vi "Assemble Process Data for Logging.vi"(8 "error in":errorcluster, 10 "Processing loop variables":T1 {"CurrInverter"."last updated" format="%<%H:%M\n%d/%m/%Y>T"; "CurrInverter"."set flag" items=["False", "True"]}) -> (0 "error out":errorcluster, 1 "MeasData":T8, 2 "Processing loop vars out":T1 {"CurrInverter"."last updated" format="%<%H:%M\n%d/%m/%Y>T"; "CurrInverter"."set flag" items=["False", "True"]})   [LabVIEW 2019, in "Main.lvclass"]
doc: "Developed by Kevin Thompson\nkevin@thompsonengineering.net\n\nCopyright 2020\nThompson Engineering, LLC"
uses:
  Main.lvclass
  Common/DataTypes/InverterPhaseData--cluster.ctl
  Common/DataQ_SE/TD MeasData--cluster.ctl
  subvis/DataTypes/averaging variables.ctl
  subvis/DataTypes/ESR alarm variables.ctl
  subvis/DataTypes/Processing loop variables--cluster.ctl
  Common/DataTypes/inverter gain range--cluster.ctl
  Common/DataTypes/inverter offset range--cluster.ctl
  Common/DataTypes/inverter info v2--cluster.ctl
  Common/DataTypes/Inverter database record v2--cluster.ctl
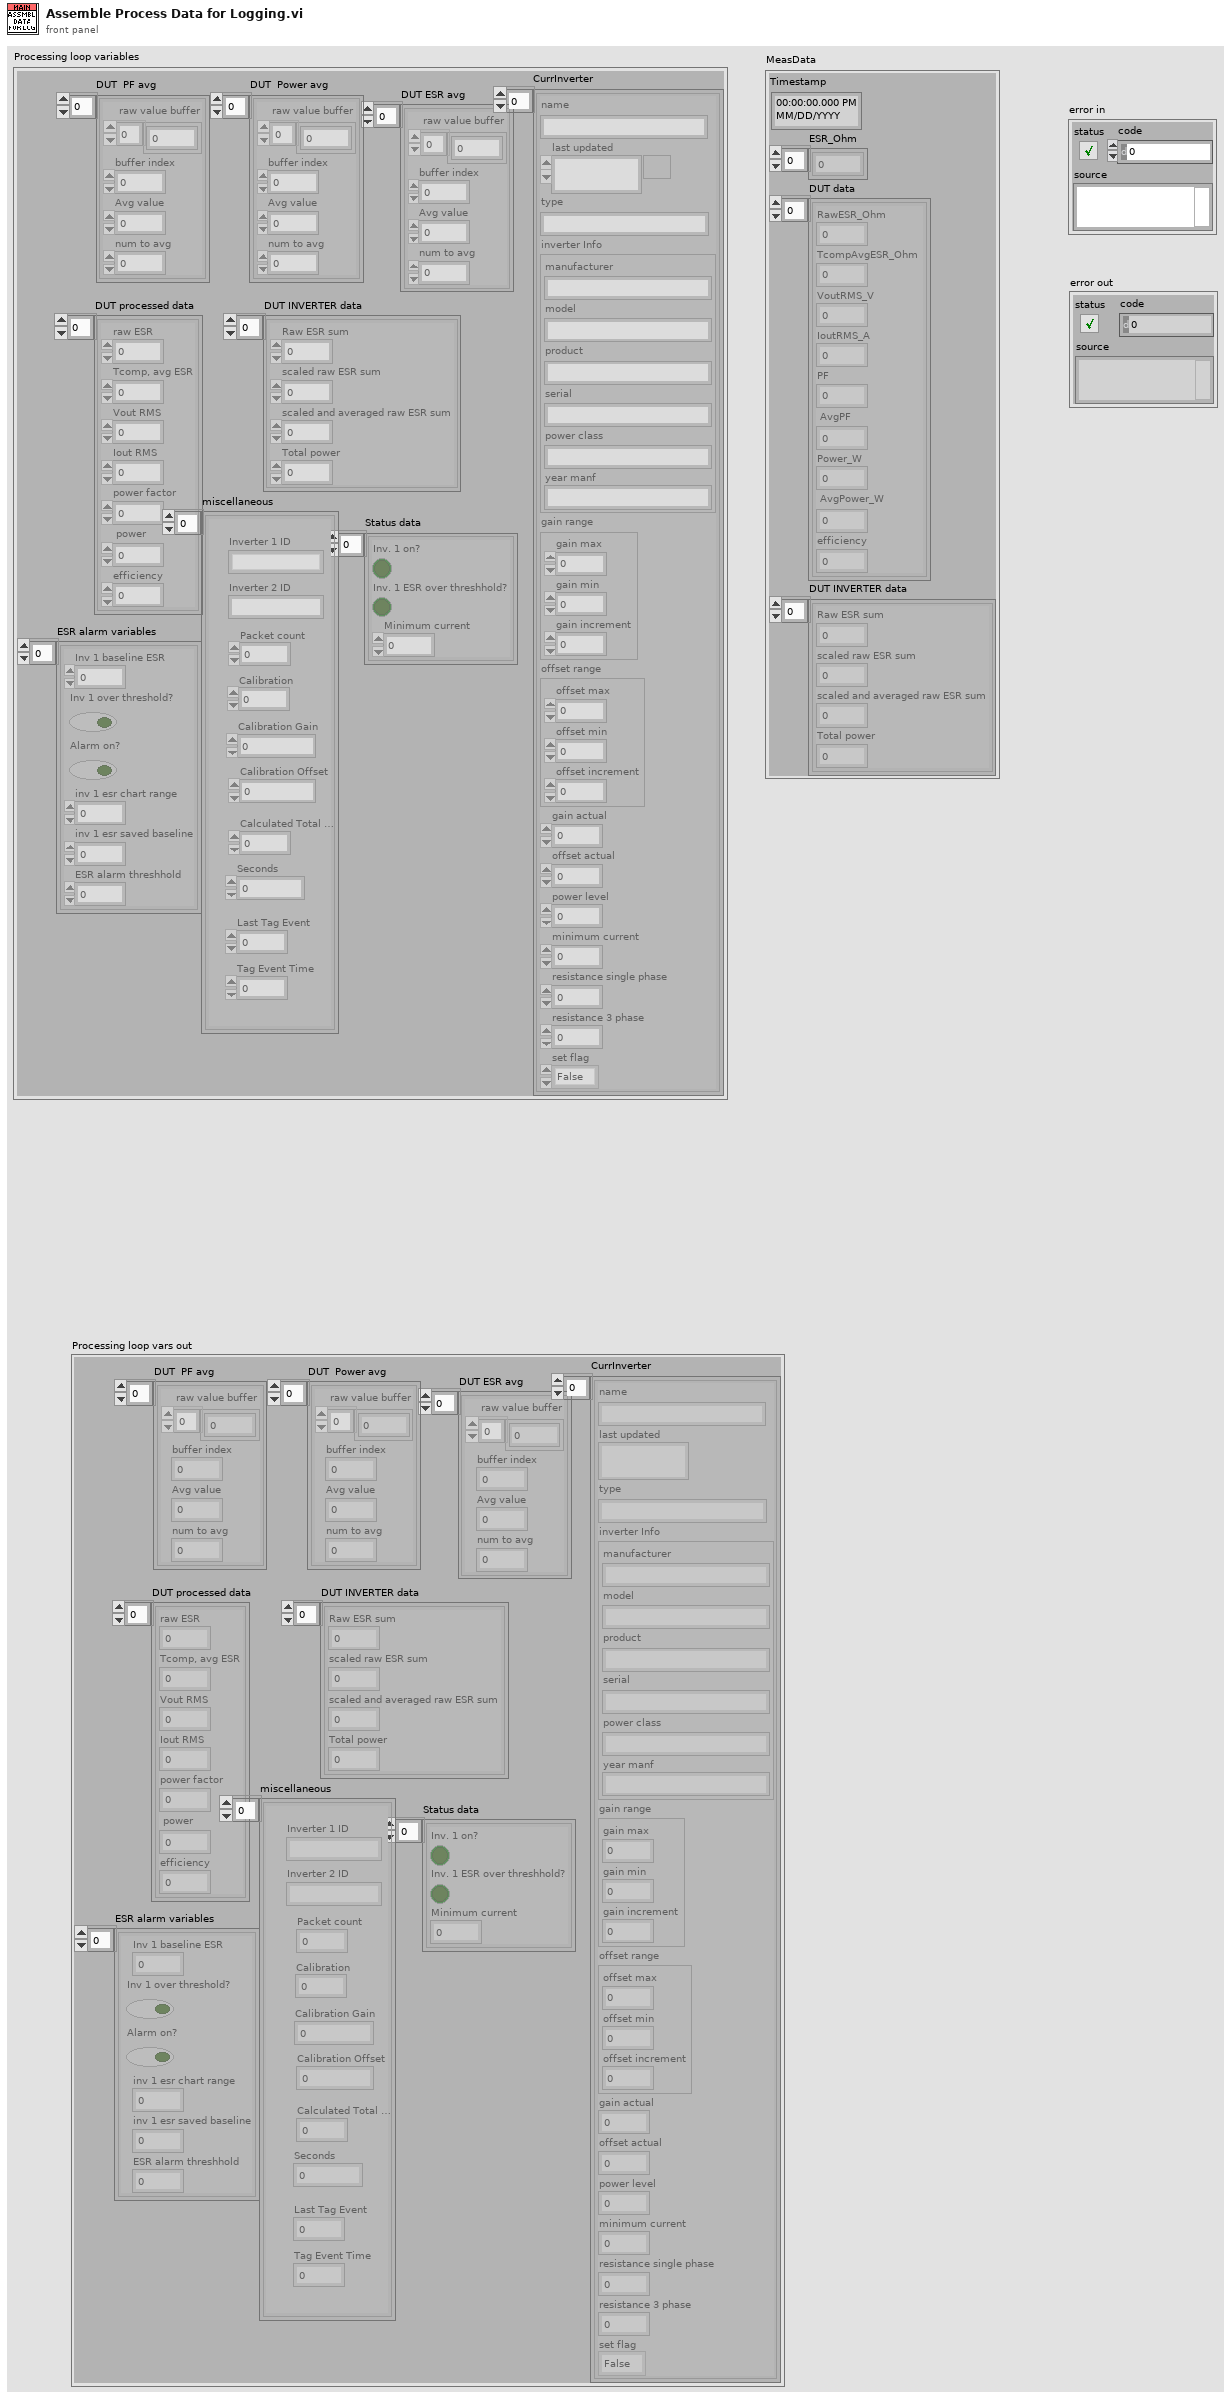
[diagram p1: front panel]
types:
  T1 = typedef "Main.lvclass/Processing loop variables--cluster.ctl" = cluster{"DUT ESR avg":T2[], "DUT  PF avg":T2[], "DUT  Power avg ":T2[], "DUT processed data":cluster{"raw ESR":dbl, "Tcomp, avg ESR":dbl, "Vout RMS":dbl, "Iout RMS":dbl, "power factor":dbl, "power":dbl, "efficiency":dbl}[], "ESR alarm variables":T3[], "Status data":cluster{"Inv. 1 on?":bool, "Inv. 1 ESR over threshhold?":bool, "Minimum current":dbl}[], "CurrInverter":T4[], "miscellaneous":cluster{"Inverter 1 ID":string, "Inverter 2 ID":string, "Packet count":u32, "Calibration":dbl, "Calibration Gain":dbl, "Calibration Offset":dbl, "Calculated Total Power":dbl, "Seconds":dbl, "Last Tag Event":dbl, "Tag Event Time":dbl}[], "DUT INVERTER data":cluster{"Raw ESR sum":dbl, "scaled raw ESR sum":dbl, "scaled and averaged raw ESR sum":dbl, "Total power":dbl}[]}
  T2 = typedef "Main.lvclass/averaging variables.ctl" = cluster{"raw value buffer":dbl[], "buffer index":i32, "Avg value":dbl, "num to avg":i32}
  T3 = typedef "Main.lvclass/ESR alarm variables.ctl" = cluster{"Inv 1 baseline ESR":dbl, "Inv 1 over threshold?":bool, "Alarm on?":bool, "inv 1 esr chart range":dbl, "inv 1 esr saved baseline":dbl, "ESR alarm threshhold":dbl}
  T4 = typedef "Inverter database record v2--cluster.ctl" = cluster{"name":string, "last updated":timestamp, "type":string, "inverter Info":T5, "gain range":T6, "offset range":T7, "gain actual":dbl, "offset actual":dbl, "power level":dbl, "minimum current":dbl, "resistance single phase":dbl, "resistance 3 phase":dbl, "set flag":u16}
  T5 = typedef "inverter info v2--cluster.ctl" = cluster{"manufacturer":string, "model":string, "product":string, "serial":string, "power class":string, "year manf":string}
  T6 = typedef "inverter gain range--cluster.ctl" = cluster{"gain max":dbl, "gain min":dbl, "gain increment":dbl}
  T7 = typedef "inverter offset range--cluster.ctl" = cluster{"offset max":dbl, "offset min":dbl, "offset increment":dbl}
  T8 = typedef "TD MeasData--cluster.ctl" = cluster{"Timestamp":timestamp, "ESR_Ohm":dbl[], "DUT data":T9[], "DUT INVERTER data":cluster{"Raw ESR sum":dbl, "scaled raw ESR sum":dbl, "scaled and averaged raw ESR sum":dbl, "Total power":dbl}[]}
  T9 = typedef "InverterPhaseData--cluster.ctl" = cluster{"RawESR_Ohm":dbl, "TcompAvgESR_Ohm":dbl, "VoutRMS_V":dbl, "IoutRMS_A":dbl, "PF":dbl, "AvgPF":dbl, "Power_W":dbl, "AvgPower_W":dbl, "efficiency":dbl}
  T10 = cluster{"raw ESR":dbl, "Tcomp, avg ESR":dbl, "Vout RMS":dbl, "Iout RMS":dbl, "power factor":dbl, "power":dbl, "efficiency":dbl}[]
  T11 = cluster{"Raw ESR sum":dbl, "scaled raw ESR sum":dbl, "scaled and averaged raw ESR sum":dbl, "Total power":dbl}[]
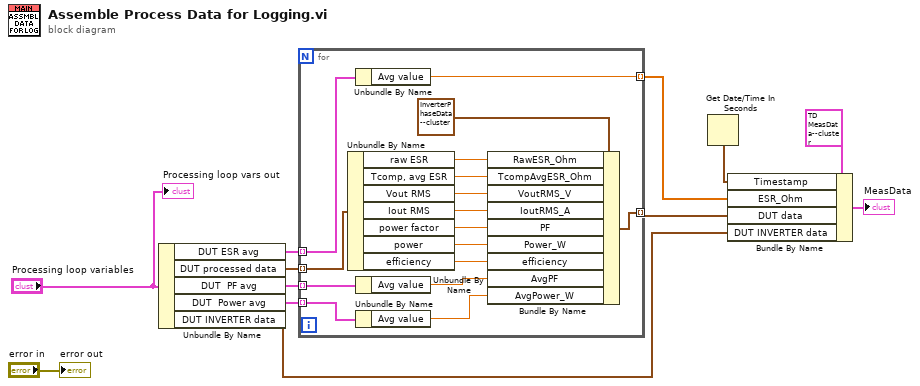
[diagram p0: block diagram]
diagram:
  n1 = Unbundle By Name("Processing loop variables") -> ("DUT ESR avg"=w1:T2[], "DUT processed data"=w4:T10, "DUT  PF avg"=w3:T2[], "DUT  Power avg"=w2:T2[], "DUT INVERTER data"=w5:T11)
  n2 = for {
    tunnel: w4 -> [w28] mode=indexing
    tunnel: w1 -> [w27] mode=indexing
    tunnel: [w26] -> w8 mode=indexing
    tunnel: [w25] -> w7 mode=indexing
    tunnel: w3 -> [w16] mode=indexing
    tunnel: w2 -> [w15] mode=indexing
    n3 = Unbundle By Name(w28) -> ("raw ESR"=w18:dbl, "Tcomp, avg ESR"=w19:dbl, "Vout RMS"=w20:dbl, "Iout RMS"=w21:dbl, "power factor"=w22:dbl, "power"=w23:dbl, "efficiency"=w24:dbl)
    n4 = Unbundle By Name(w27) -> ("Avg value"=w26:dbl)
    n5 = Unbundle By Name(w16) -> ("Avg value"=w13:dbl)
    n6 = Unbundle By Name(w15) -> ("Avg value"=w14:dbl)
    n7 = Bundle By Name(cluster=T9 {"RawESR_Ohm"=0.0, "TcompAvgESR_Ohm"=0.0, "VoutRMS_V"=0.0, "IoutRMS_A"=0.0, "PF"=0.0, "AvgPF"=0.0, "Power_W"=0.0, "AvgPower_W"=0.0, "efficiency"=0.0} ("Phase3 Data"), "RawESR_Ohm"=w18, "TcompAvgESR_Ohm"=w19, "VoutRMS_V"=w20, "IoutRMS_A"=w21, "PF"=w22, "Power_W"=w23, "efficiency"=w24, "AvgPF"=w13, "AvgPower_W"=w14) -> (w25:T9)
  }
  n8 = Get Date/Time In Seconds() -> (seconds since 1Jan1904=w10:timestamp)
  n9 = Bundle By Name(cluster=T8 {"Timestamp"=timestamp(0 s since 1904-01-01), "ESR_Ohm"=[], "DUT data"=[], "DUT INVERTER data"=[]} ("MeasData"), "Timestamp"=w10, "ESR_Ohm"=w8, "DUT data"=w7, "DUT INVERTER data"=w5) -> (→"MeasData":T8)
  "error out" <- "error in"
  "Processing loop vars out" <- "Processing loop variables"
